vi "NIMS_DF_fir_linf(m, f, mag, ripple, tm).vi"(7 "type":T1(ring), 8 "ripple":dbl[](array[numeric]), 9 "mag":dbl[](array[numeric]), 10 "f":dbl[](array[numeric]), 11 "flag":enum32{"minorder"}(ring)) -> (0 "error":i32, 3 "b":dbl[](array[numeric]))   [LabVIEW 2017, in "NI_DigFilter_MathScript.lvlib"]
uses:
  <vilib>/addons/Digital Filter Design/NI_DigFilter_MathScript.lvlib
  <vilib>/addons/Digital Filter Design/_REMEZ.llb/remez_fir filter type.ctl
  <vilib>/addons/Digital Filter Design/NI_DigFilterLicensed.lvlib
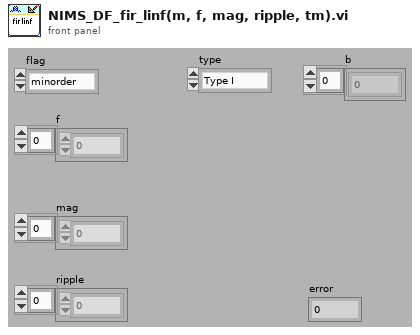
[diagram p1: front panel]
types:
  T1 = enum32{"Type I", "Type II", "Type III", "Type IV"}
  T2 = typedef "NI_DigFilterLicensed.lvlib/remez_fir filter type.ctl" = enum32{"Symmetric", "Antisymmetric", "Differentiator", "Hilbert", "Minimum Phase", "Maximum Phase"}
  T3 = typedef "NI_DigFilterLicensed.lvlib/DFD Adv Band Spec.ctl" = cluster{"band specification":cluster{"freq":dbl, "amplitude":dbl, "weight":dbl}[], "ripple constraint":dbl}
  T4 = typedef "NI_DigFilterLicensed.lvlib/DFD Filter Obj.ctl" = cluster{"mSRate_Fs":dbl, "mSRate_Version":string, "mSRate_Comments":string, "mSRate_OrgCoef":T5, "mSRate_CurCoef":T5, "mSRate_Quantized?":bool, "mSRate_QCoef":T5, "mSRate_QSettings":T7[], "mSRate_Order":i32, "mSRate_Scaling":cluster{"mSRate_ScaleByPowerOf2?":bool, "mSRate_ScaleType":T9}}
  T5 = typedef "NI_DigFilterLicensed.lvlib/DFD Filter Coef.ctl" = cluster{"type":T6, "gain":dbl, "coef a (k)":dbl[], "coef b (v)":dbl[]}
  T6 = typedef "NI_DigFilterLicensed.lvlib/DFD Filter Structure Type Selector.ctl" = enum16{"Undefined", "FIR Direct Form", "FIR Direct Form Transposed", "FIR Symmetric", "FIR Antisymmetric", "IIR Direct Form I", "IIR Direct Form I Transposed", "IIR Direct Form II", "IIR Direct Form II Transposed", "IIR Cascaded Second Order Sections Form I", "IIR Cascaded Second Order Sections Form I Transposed", "IIR Cascaded Second Order Sections Form II", "IIR Cascaded Second Order Sections Form II Transposed", "Lattice Allpass (basic sections)", "Lattice Allpass (one multiplier sections)", "Lattice Allpass (normalized sections)", "Lattice AR (basic sections)", "Lattice AR (one multiplier sections)", "Lattice AR (normalized sections)", "Lattice MA (minimum phase)", "Lattice MA (maximum phase)", "Lattice ARMA (basic sections)", "Lattice ARMA (one multiplier sections)", "Lattice ARMA (normalized sections)"}
  T7 = typedef "NI_DigFilterLicensed.lvlib/dfd_Internal Quantization Settings.ctl" = cluster{"source":T8, "wl":i16, "iwl":i16, "overflow mode":enum16{"Saturation", "Wrap"}, "rounding mode":enum16{"Nearest", "Truncation"}, "signed?":bool}
  T8 = typedef "NI_DigFilterLicensed.lvlib/dfd_Internal Quantization Srcs.ctl" = u16
  T9 = typedef "NI_DigFilterLicensed.lvlib/DFD Coef Norm Type.ctl" = enum16{"No Norm", "Time Domain 1-Norm", "Time Domain 2-Norm", "Time Domain Inf-Norm"}
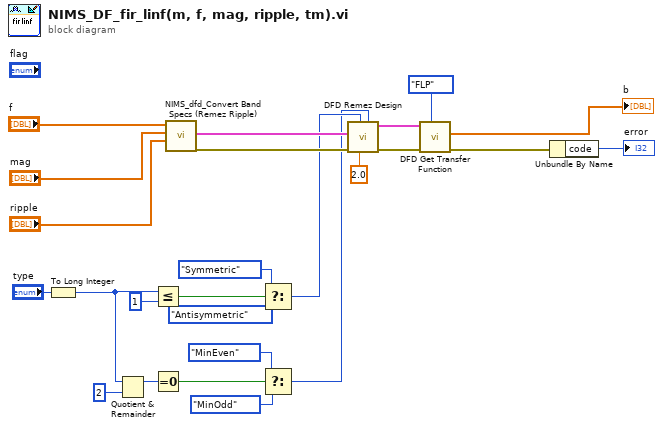
[diagram p0: block diagram]
diagram:
  n1 = To Long Integer(number="type") -> (32bit integer=w21:i32)
  n2 = Quotient & Remainder(x=w21, y=2) -> (x-y*floor(x/y)=w13:i32)  [unwired: 1 out]
  n3 = Less Or Equal?(x=w21, y=1) -> (x <= y?=w12:bool)
  n4 = Equal To 0?(x=w13) -> (x = 0?=w9:bool)
  n5 = call <vilib>:"NIMS_dfd_Convert Band Specs (Remez Ripple).vi"("Ripple"="ripple", "A"="mag", "F"="f") -> ("error out"=w16:errorcluster, "band specs"=w17:T3[])  [unwired: 7 out]
  n6 = Select(t=remez_fir_filter_type."Symmetric" ("filter type"), s=w12, f=remez_fir_filter_type."Antisymmetric" ("filter type")) -> (s? t:f=w8:T2)
  n7 = Select(t=enum32{"User Defined", "MinEven", "MinOdd"}."MinEven" ("minimum order"), s=w9, f=enum32{"User Defined", "MinEven", "MinOdd"}."MinOdd" ("minimum order")) -> (s? t:f=w7:enum32{"User Defined", "MinEven", "MinOdd"})
  n8 = call <vilib>:"DFD Remez Design.vi"("minimum order"=w7, "fs [Hz]"=2.0, "filter type"=w8, "error in (no error)"=w16, "band specs"=w17) -> ("error out"=w2:errorcluster, "filter out"=w3:T4)  [unwired: 2 in, 3 out]
  n9 = call <vilib>:"DFD Get Transfer Function.vi"("type (FLP)"=enum16{"FLP", "FXP"}."FLP", "error in (no error)"=w2, "filter in"=w3) -> ("error out"=w20:errorcluster, "numerator"=→"b":dbl[])  [unwired: 7 out]
  n10 = Unbundle By Name(w20) -> ("code"=→"error":i32)
